vi "VisualizationManager.vi"(7 "Action":T1, 8 "error in (no error)":errorcluster, 9 "Load In SubPanel?":bool, 10 "Module Name":string, 11 "Open Visualization VIs in":T2[](array[typedef])) -> (0 "error out":errorcluster, 1 "In SubPanel?":bool, 2 "Module Name out":string, 3 "Open Visualization VIs out":T2[](array[typedef]))   [LabVIEW 2018]
uses:
  OpenVisualizationVIs.ctl
  VisualizationManagerActions.ctl
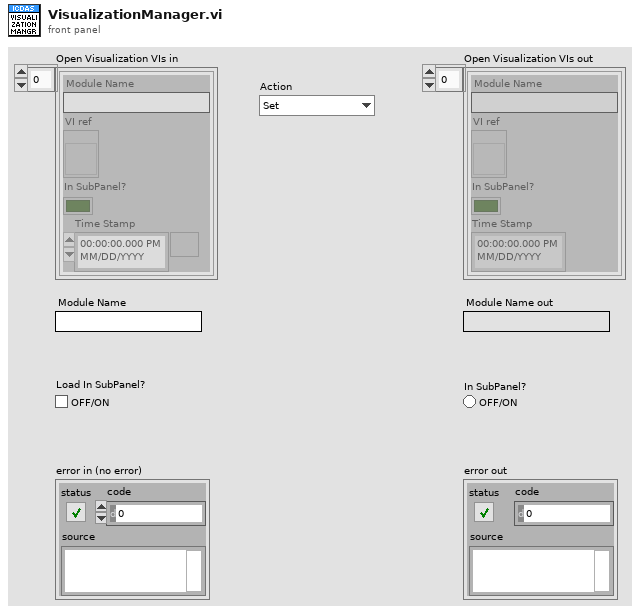
[diagram p1: front panel]
types:
  T1 = typedef "VisualizationManagerActions.ctl" = enum16{"Set", "LoadModVI", "PopInOutModVI", "Add", "Clear", "CloseVisMod", "LoadLatestModule", "Get"}
  T2 = typedef "OpenVisualizationVIs.ctl" = cluster{"Module Name":string, "VI ref":refnum<vi>, "In SubPanel?":bool, "Time Stamp":timestamp}
  T3 = enum32{"Invalid", "Standard", "Closed", "Hidden", "Minimized", "Maximized"}
  T4 = typedef "cntlRefs.ctl" = cluster{"rngFGen":refnum<vi>, "rngDigitizer":refnum<vi>, "btnHide":refnum<vi>, "rngInst":refnum<vi>, "PluginTree":refnum<vi>, "TestListboxRef":refnum<vi>, "path.tstFile":refnum<vi>, "cmbxRunningModules":refnum<vi>, "TestDataSubPanel":refnum<vi>, "TestDataCaption":refnum<vi>, "btnPopInOut":refnum<vi>, "PluginMgrQ":refnum<queue>, "TestMgrQ":refnum<queue>, "TestMgrSubPanel":refnum<vi>, "PluginMgrSubPanel":refnum<vi>, "PwrReqHandle":u32, "btnStopOneTest":refnum<vi>, "pathUserfiles":refnum<vi>, "PluginTreeCaption":refnum<vi>, "MainVIRef":refnum<vi>, "btnStatus":refnum<vi>}
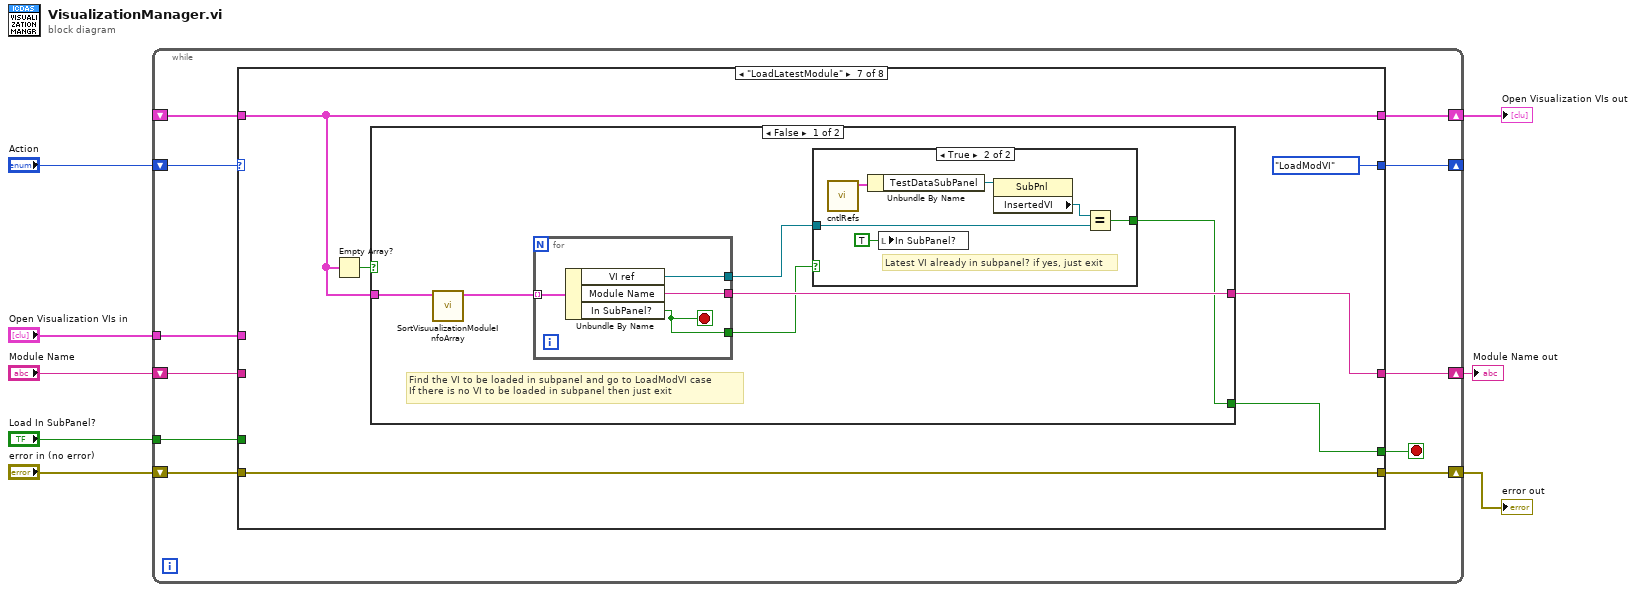
[diagram p0: block diagram]
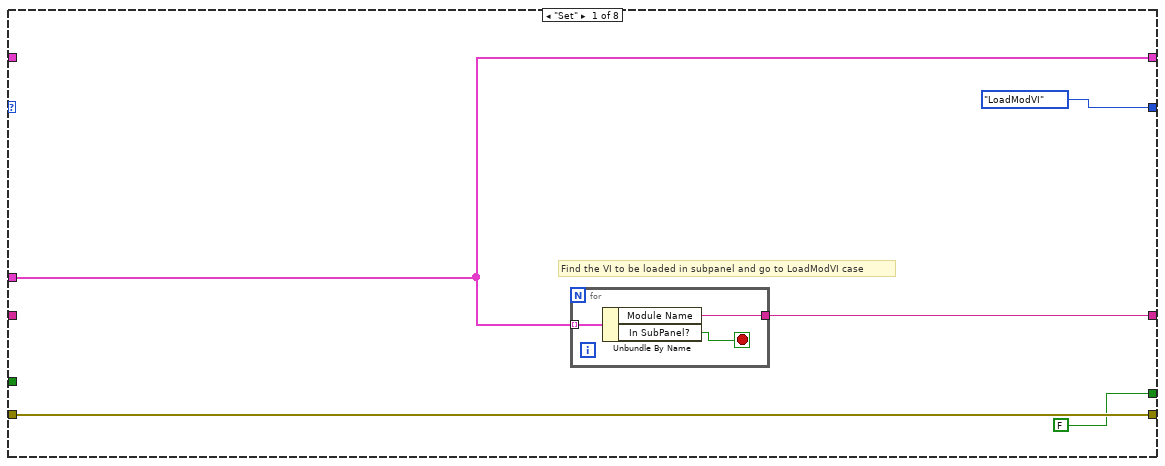
[diagram p2: hidden frame]
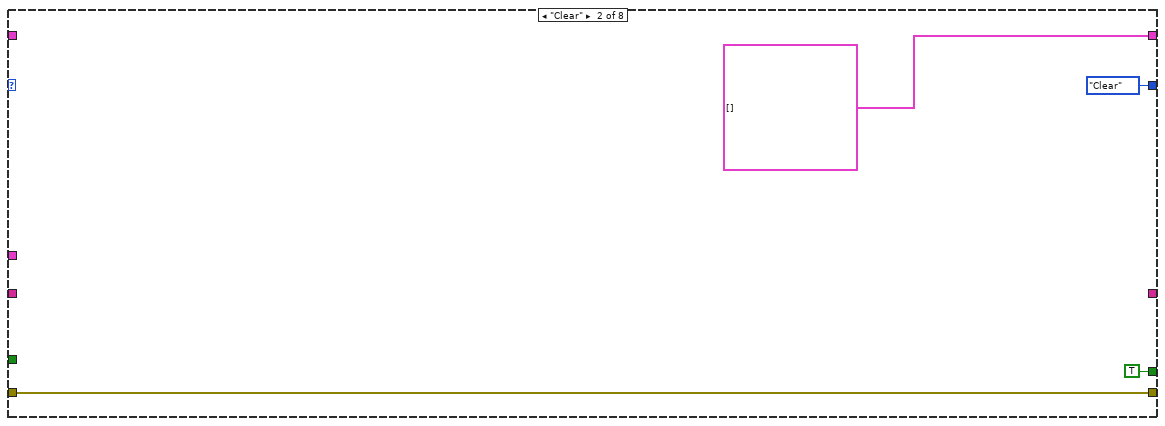
[diagram p3: hidden frame]
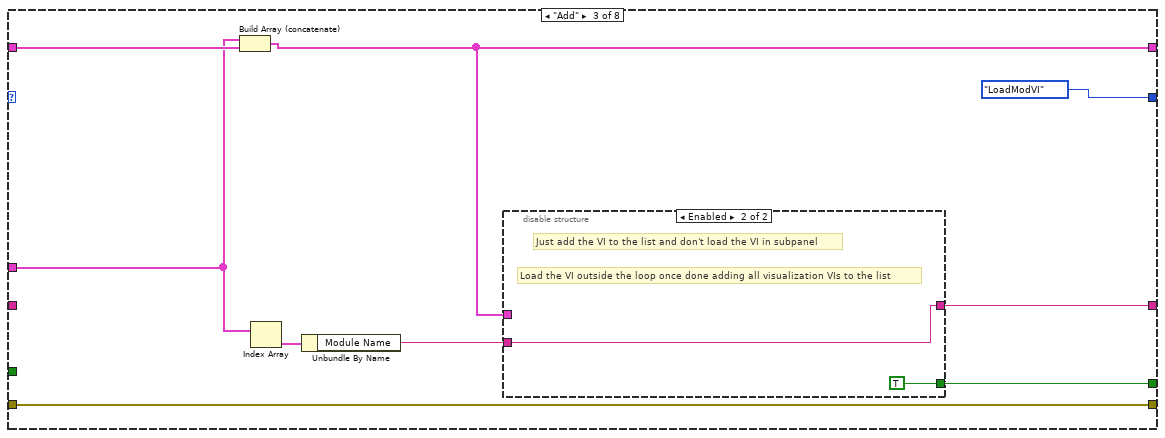
[diagram p4: hidden frame]
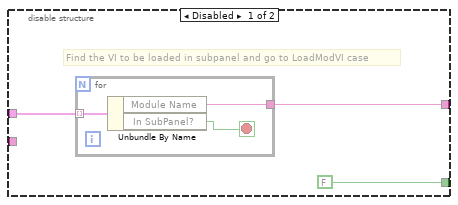
[diagram p5: hidden frame]
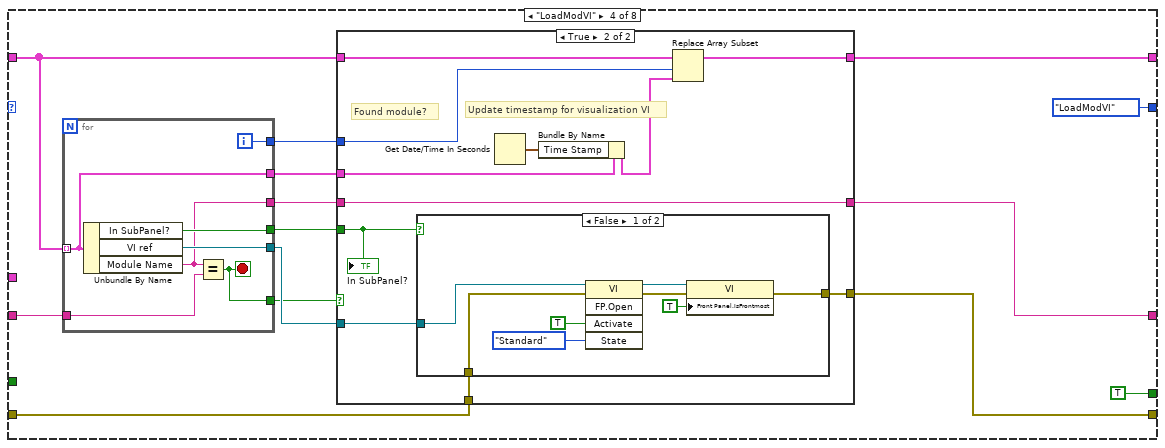
[diagram p6: hidden frame]
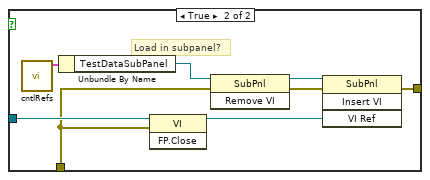
[diagram p8: hidden frame]
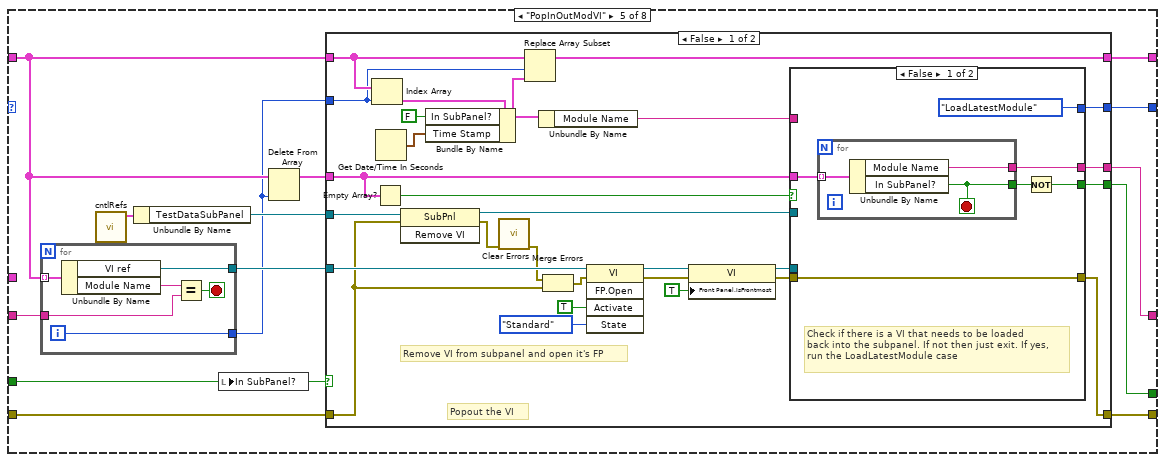
[diagram p9: hidden frame]
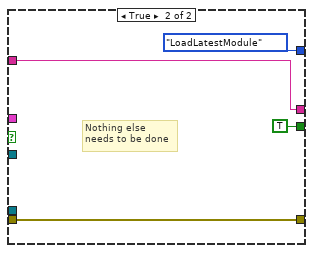
[diagram p10: hidden frame]
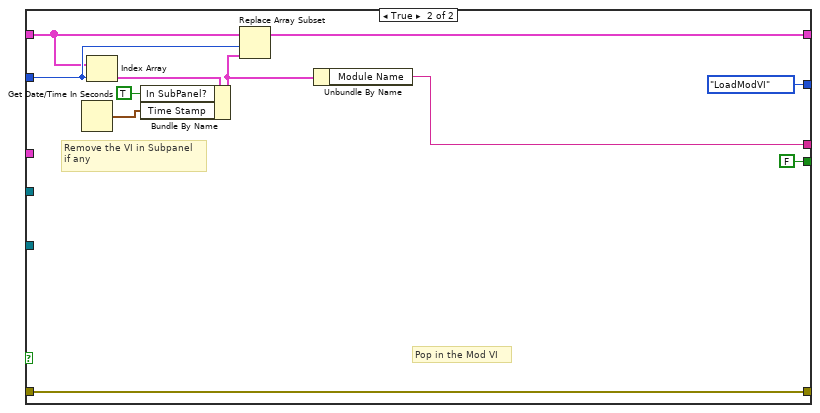
[diagram p11: hidden frame]
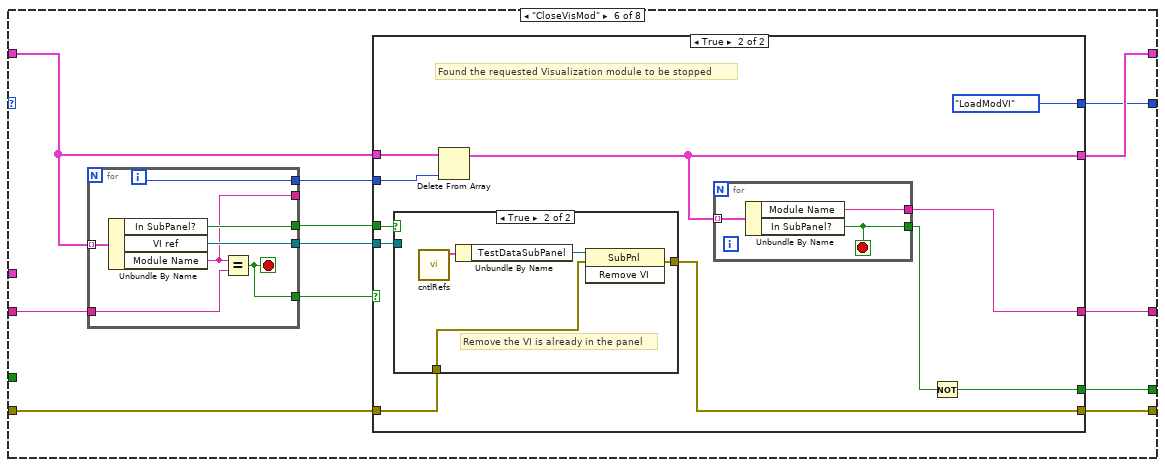
[diagram p12: hidden frame]
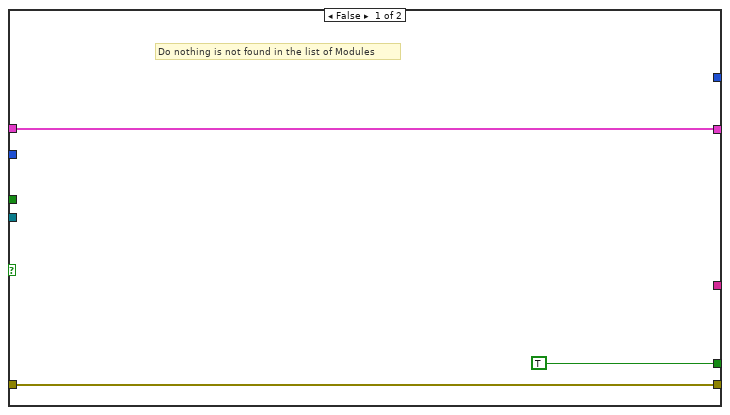
[diagram p13: hidden frame]
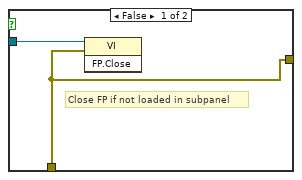
[diagram p14: hidden frame]
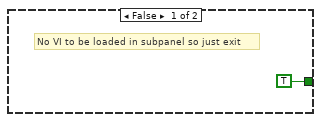
[diagram p15: hidden frame]
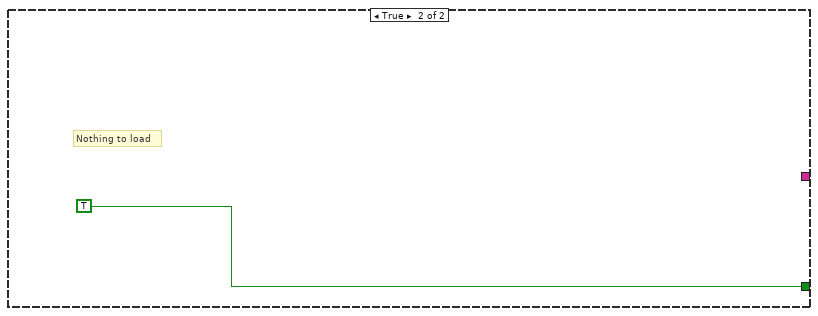
[diagram p16: hidden frame]
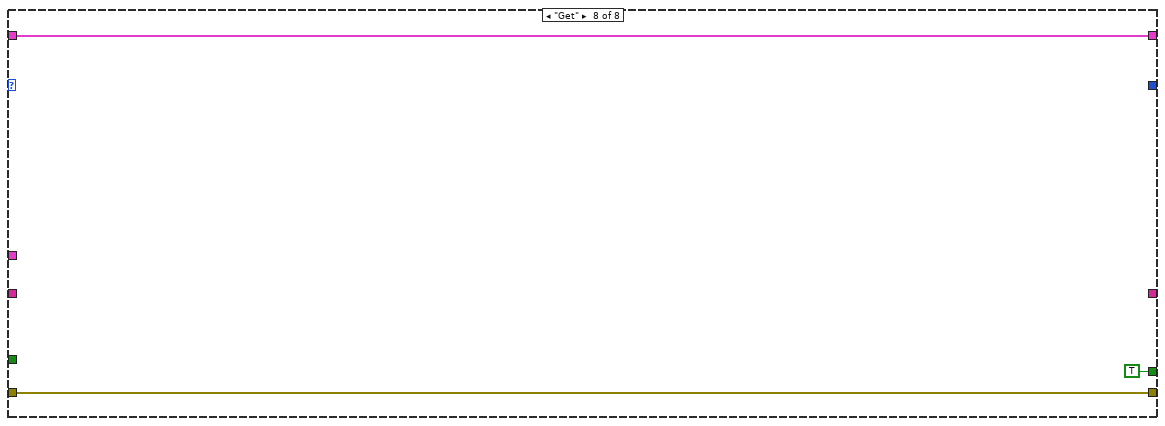
[diagram p17: hidden frame]
diagram:
  n1 = while {
    tunnel: "Load In SubPanel?" -> [w13]
    shift-right: [w19] -> w8
    shift-left: "error in (no error)" -> [w18]
    tunnel: "Open Visualization VIs in" -> [w16]
    shift-right: [w15] -> w4
    shift-left: _ -> [w11]
    shift-right: [w10] -> _
    shift-left: "Action" -> [w14]
    shift-right: [w9] -> w1
    shift-left: "Module Name" -> [w17]
    stop <- w12 stop-if-true
    n2 = case shown="\"LoadLatestModule\"" w14 {
      tunnel: w16 -> [w22 _ w34 _ _ _ _ _]
      tunnel: [w22 T2[] [] ("Open Visualization VIs in") w35 w49 w100 w179 w213 w239] -> w15
      tunnel: w11 -> [_ _ w36 w51 w102 w171 w213 w239]
      tunnel: w17 -> [_ _ _ w62 w108 w182 _ _]
      tunnel: w18 -> [w24 w31 w40 w60 w109 w173 w216 w238]
      tunnel: [w24 w31 w40 w59 w110 w172 w216 w238] -> w19
      tunnel: w13 -> [_ _ _ _ w99 _ _ _]
      tunnel: [FALSE TRUE w37 TRUE w104 w176 w215 TRUE] -> w12
      tunnel: [VisualizationManagerActions."LoadModVI" ("Action") VisualizationManagerActions."Clear" ("Action") VisualizationManagerActions."LoadModVI" ("Action") VisualizationManagerActions."LoadModVI" ("Action") w105 w175 VisualizationManagerActions."LoadModVI" ("Action") _] -> w10
      tunnel: [w21 _ w38 w53 w103 w174 w217 _] -> w9
      frame "Set" {
        # "Find the VI to be loaded in subpanel and go to LoadModVI case"
        n3 = for {
          tunnel: w22 -> [w27] mode=indexing
          tunnel: [w26] -> w21
          stop <- w25 stop-if-true
          n4 = Unbundle By Name(w27) -> ("Module Name"=w26:string, "In SubPanel?"=w25:bool)
        }
      }
      frame "Clear" {
      }
      frame "Add" {
        n5 = Build Array (concatenate)(w34, w36) -> (w35:T2[])
        n6 = Index Array(array=w34) -> (element=w33:T2)  [unwired: 1 in]
        n7 = Unbundle By Name(w33) -> ("Module Name"=w32:string)
        n8 = disable-structure shown="Enabled" {
          disable-tunnel: [w43 w47] -> w38
          disable-tunnel: [FALSE TRUE] -> w37
          disable-tunnel: w35 -> [w41 _]
          disable-tunnel: w32 -> [_ w47]
          frame Disabled {
            # "Find the VI to be loaded in subpanel and go to LoadModVI case"
            n9 = for {
              tunnel: w41 -> [w46] mode=indexing
              tunnel: [w45] -> w43
              stop <- w44 stop-if-true
              n10 = Unbundle By Name(w46) -> ("Module Name"=w45:string, "In SubPanel?"=w44:bool)
            }
          }
          frame Enabled {
            # "Load the VI outside the loop once done adding all visualization VIs to the list"
            # "Just add the VI to the list and don't load the VI in subpanel"
          }
        }
      }
      frame "LoadModVI" {
        n11 = for {
          tunnel: w51 -> [w93] mode=indexing
          tunnel: w62 -> [w98]
          tunnel: [w97] -> w61
          tunnel: [w96] -> w58
          tunnel: [w95] -> w57
          tunnel: [w94] -> w54
          tunnel: [w93] -> w50
          tunnel: [w92] -> w52
          i -> [w92]
          stop <- w96 stop-if-true
          n12 = Unbundle By Name(w93) -> ("In SubPanel?"=w95:bool, "VI ref"=w97:refnum<vi>, "Module Name"=w94:string)
          n13 = Equal?(x=w94, y=w98) -> (x = y?=w96:bool)
        }
        n14 = case shown="True" w58 {
          tunnel: w61 -> [_ w76]
          tunnel: w60 -> [w65 w75]
          tunnel: [w65 w74] -> w59
          tunnel: w57 -> [_ w73]
          tunnel: w54 -> [w64 w72]
          tunnel: [w64 w72] -> w53
          tunnel: w52 -> [_ w70]
          tunnel: w51 -> [w63 w71]
          tunnel: w50 -> [_ w69]
          tunnel: [w63 w66] -> w49
          frame False {
          }
          frame True {
            # "Update timestamp for visualization VI"
            # "Found module?"
            n15 = case shown="False" w73 {
              tunnel: w76 -> [w82 w91]
              tunnel: w75 -> [w81 w85]
              tunnel: [w79 w90] -> w74
              frame False {
                n16 = invoke class="VI" method="FP.Open"(reference=w82, error in=w81, "Activate"=TRUE ("Activate?"), "State"=T3."Standard") -> (reference out=w78:refnum<vi>, error out=w80:errorcluster)  [unwired: 1 in, 3 out]
                n17 = property class="VI"(reference=w78, error in=w80, "Front Panel.IsFrontmost"=TRUE ("Front Panel Window:Is Frontmost")) -> (error out=w79:errorcluster)  [unwired: 1 out]
              }
              frame True {
                # "Load in subpanel?"
                n18 = call "cntlRefs.vi"() -> ("cntlRefs"=w88:T4)  [unwired: 10 in, 1 out]
                n19 = Unbundle By Name(w88) -> ("TestDataSubPanel"=w86:refnum<vi>)
                n20 = invoke class="VI" method="FP.Close"(reference=w91, error in=w85) -> (reference out=w87:refnum<vi>)  [unwired: 1 in, 2 out]
                n21 = invoke class="SubPnl" method="Remove VI"(reference=w86) -> (reference out=w89:refnum<vi>)  [unwired: 2 in, 2 out]
                n22 = invoke class="SubPnl" method="Insert VI"(reference=w89, error in=w85, "VI Ref"=w87) -> (error out=w90:errorcluster)  [unwired: 1 in, 3 out]
              }
            }
            n23 = Get Date/Time In Seconds() -> (seconds since 1Jan1904=w67:timestamp)
            n24 = Bundle By Name(cluster=w69, "Time Stamp"=w67) -> (w68:T2)
            n25 = Replace Array Subset(array=w71, new element=w68, index=w70) -> (w66:T2[])
            "In SubPanel?" <- w73
          }
        }
      }
      frame "PopInOutModVI" {
        n26 = for {
          tunnel: w102 -> [w170] mode=indexing
          tunnel: w108 -> [w168]
          tunnel: [w166] -> w107
          tunnel: [w165] -> w101
          i -> [w165]
          stop <- w167 stop-if-true
          n27 = Unbundle By Name(w170) -> ("VI ref"=w166:refnum<vi>, "Module Name"=w169:string)
          n28 = Equal?(x=w169, y=w168) -> (x = y?=w167:bool)
        }
        n29 = call "cntlRefs.vi"() -> ("cntlRefs"=w111:T4)  [unwired: 10 in, 1 out]
        n30 = Unbundle By Name(w111) -> ("TestDataSubPanel"=w112:refnum<vi>)
        n31 = local write "In SubPanel?"(w99) -> ()
        n32 = Delete From Array(array=w102, index=w101) -> (array with subset deleted=w106:T2[])  [unwired: 1 in, 1 out]
        n33 = case shown="False" w99 {
          tunnel: w112 -> [w140 _]
          tunnel: [w127 w155] -> w110
          tunnel: w109 -> [w130 w155]
          tunnel: w107 -> [w137 _]
          tunnel: w106 -> [w135 _]
          tunnel: [w128 VisualizationManagerActions."LoadModVI" ("Action")] -> w105
          tunnel: [w126 FALSE] -> w104
          tunnel: [w125 w156] -> w103
          tunnel: w102 -> [w124 w161]
          tunnel: w101 -> [w121 w162]
          tunnel: [w123 w160] -> w100
          frame False {
            # "Remove VI from subpanel and open it's FP"
            # "Popout the VI"
            n34 = Index Array(array=w124, index=w121) -> (element=w122:T2)
            n35 = Empty Array?(array=w135) -> (empty?=w136:bool)
            n36 = Get Date/Time In Seconds() -> (seconds since 1Jan1904=w117:timestamp)
            n37 = invoke class="SubPnl" method="Remove VI"(reference=w140, error in=w130) -> (reference out=w133:refnum<vi>, error out=w132:errorcluster)  [unwired: 1 in, 1 out]
            n38 = Bundle By Name(cluster=w122, "In SubPanel?"=FALSE, "Time Stamp"=w117) -> (w119:T2)
            n39 = call <vilib>:"Clear Errors.vi"("error in (no error)"=w132) -> ("error out"=w131:errorcluster)  [unwired: 5 in, 1 out]
            n40 = Replace Array Subset(array=w124, new element=w119, index=w121) -> (w123:T2[])
            n41 = Unbundle By Name(w119) -> ("Module Name"=w118:string)
            n42 = Merge Errors(w131, w130) -> (w129:errorcluster)
            n43 = invoke class="VI" method="FP.Open"(reference=w137, error in=w129, "Activate"=TRUE ("Activate?"), "State"=T3."Standard") -> (reference out=w115:refnum<vi>, error out=w134:errorcluster)  [unwired: 1 in, 3 out]
            n44 = property class="VI"(reference=w115, error in=w134, "Front Panel.IsFrontmost"=TRUE ("Front Panel Window:Is Frontmost")) -> (reference out=w114:refnum<vi>, error out=w116:errorcluster)
            n45 = case shown="False" w136 {
              tunnel: w135 -> [w145 _]
              tunnel: w116 -> [w144 w153]
              tunnel: w133 -> [_ _]
              tunnel: [VisualizationManagerActions."LoadLatestModule" ("Action") VisualizationManagerActions."LoadLatestModule" ("Action")] -> w128
              tunnel: [w144 w153] -> w127
              tunnel: [w142 TRUE] -> w126
              tunnel: [w141 w150] -> w125
              tunnel: w118 -> [_ w150]
              tunnel: w114 -> [_ _]
              frame False {
                # "Check if there is a VI that needs to be loaded\nback into the subpanel. If not then just exit. If yes,\nrun the LoadLatestModule case"
                n46 = for {
                  tunnel: w145 -> [w149] mode=indexing
                  tunnel: [w148] -> w141
                  tunnel: [w147] -> w143
                  stop <- w147 stop-if-true
                  n47 = Unbundle By Name(w149) -> ("Module Name"=w148:string, "In SubPanel?"=w147:bool)
                }
                n48 = Not(x=w143) -> (.not. x?=w142:bool)
              }
              frame True {
                # "Nothing else\nneeds to be done"
              }
            }
          }
          frame True {
            # "Remove the VI in Subpanel\nif any"
            # "Pop in the Mod VI"
            n49 = Get Date/Time In Seconds() -> (seconds since 1Jan1904=w154:timestamp)
            n50 = Index Array(array=w161, index=w162) -> (element=w164:T2)
            n51 = Bundle By Name(cluster=w164, "In SubPanel?"=TRUE, "Time Stamp"=w154) -> (w157:T2)
            n52 = Replace Array Subset(array=w161, new element=w157, index=w162) -> (w160:T2[])
            n53 = Unbundle By Name(w157) -> ("Module Name"=w156:string)
          }
        }
      }
      frame "CloseVisMod" {
        n54 = for {
          tunnel: w171 -> [w212] mode=indexing
          tunnel: w182 -> [w211]
          tunnel: [w210] -> w177
          tunnel: [w209] -> w181
          tunnel: [w208] -> w178
          tunnel: [w207] -> _
          tunnel: [w206] -> w180
          i -> [w206]
          stop <- w209 stop-if-true
          n55 = Unbundle By Name(w212) -> ("In SubPanel?"=w208:bool, "VI ref"=w210:refnum<vi>, "Module Name"=w207:string)
          n56 = Equal?(x=w207, y=w211) -> (x = y?=w209:bool)
        }
        n57 = case shown="True" w181 {
          tunnel: w171 -> [w185 w196]
          tunnel: w180 -> [_ w193]
          tunnel: [w185 w192] -> w179
          tunnel: w178 -> [_ w195]
          tunnel: w177 -> [_ w194]
          tunnel: [TRUE w190] -> w176
          tunnel: [_ VisualizationManagerActions."LoadModVI" ("Action")] -> w175
          tunnel: [_ w188] -> w174
          tunnel: w173 -> [w183 w186]
          tunnel: [w183 w187] -> w172
          frame False {
            # "Do nothing is not found in the list of Modules"
          }
          frame True {
            # "Found the requested Visualization module to be stopped"
            n58 = case shown="True" w195 {
              tunnel: w194 -> [w201 _]
              tunnel: w186 -> [w200 w203]
              tunnel: [w200 w202] -> w187
              frame False {
                # "Close FP if not loaded in subpanel"
                n59 = invoke class="VI" method="FP.Close"(reference=w201, error in=w200) -> ()  [unwired: 1 in, 3 out]
              }
              frame True {
                # "Remove the VI is already in the panel"
                n60 = call "cntlRefs.vi"() -> ("cntlRefs"=w205:T4)  [unwired: 10 in, 1 out]
                n61 = Unbundle By Name(w205) -> ("TestDataSubPanel"=w204:refnum<vi>)
                n62 = invoke class="SubPnl" method="Remove VI"(reference=w204, error in=w203) -> (error out=w202:errorcluster)  [unwired: 1 in, 2 out]
              }
            }
            n63 = Delete From Array(array=w196, index=w193) -> (array with subset deleted=w192:T2[])  [unwired: 1 in, 1 out]
            n64 = for {
              tunnel: w192 -> [w199] mode=indexing
              tunnel: [w198] -> w188
              tunnel: [w197] -> w191
              stop <- w197 stop-if-true
              n65 = Unbundle By Name(w199) -> ("Module Name"=w198:string, "In SubPanel?"=w197:bool)
            }
            n66 = Not(x=w191) -> (.not. x?=w190:bool)
          }
        }
      }
      frame "LoadLatestModule" {
        n67 = Empty Array?(array=w213) -> (empty?=w214:bool)
        n68 = case shown="False" w214 {
          tunnel: w213 -> [w223 _]
          tunnel: [w224 _] -> w217
          tunnel: [w219 TRUE] -> w215
          frame False {
            # "Find the VI to be loaded in subpanel and go to LoadModVI case\nIf there is no VI to be loaded in subpanel then just exit"
            n69 = call "SortVisuualizationModuleInfoArray.vi"("Open Visualization VIs in"=w223) -> ("Array"=w222:T2[])  [unwired: 10 in]
            n70 = for {
              tunnel: w222 -> [w235] mode=indexing
              tunnel: [w234] -> w224
              tunnel: [w233] -> w220
              tunnel: [w232] -> w221
              stop <- w233 stop-if-true
              n71 = Unbundle By Name(w235) -> ("VI ref"=w232:refnum<vi>, "Module Name"=w234:string, "In SubPanel?"=w233:bool)
            }
            n72 = case shown="True" w220 {
              tunnel: w221 -> [_ w228]
              tunnel: [TRUE w227] -> w219
              frame False {
                # "No VI to be loaded in subpanel so just exit"
              }
              frame True {
                # "Latest VI already in subpanel? if yes, just exit"
                n73 = call "cntlRefs.vi"() -> ("cntlRefs"=w231:T4)  [unwired: 10 in, 1 out]
                n74 = Unbundle By Name(w231) -> ("TestDataSubPanel"=w230:refnum<vi>)
                n75 = local write "In SubPanel?"(TRUE ("In SubPanel?")) -> ()
                n76 = property class="SubPnl"(reference=w230) -> ("InsertedVI"=w229:refnum<vi>)  [unwired: 1 in, 2 out]
                n77 = Equal?(x=w229, y=w228) -> (x = y?=w227:bool)
              }
            }
          }
          frame True {
            # "Nothing to load"
          }
        }
      }
      frame "Get" {
      }
    }
  }
  "error out" <- w8
  "Open Visualization VIs out" <- w4
  "Module Name out" <- w1
